vi "Turret Limelight Jog.vi"(11 "Jog Amount":dbl) -> ()   [LabVIEW 2019]
doc: "This template is useful for immediate subsystem actions that do not need deadband filtering\n\nBe sure to right-click and select New from Template and save with a new command name."
uses:
  SynchronousVIs/LL Offsets.vi
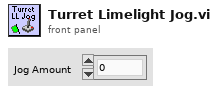
[diagram p1: front panel]
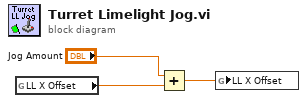
[diagram p0: block diagram]
diagram:
  n1 = global read "LL Offsets.vi" "LL X Offset"() -> (w3:dbl)
  n2 = Add(x="Jog Amount", y=w3) -> (x+y=w1:dbl)
  n3 = global write "LL Offsets.vi" "LL X Offset"(w1) -> ()
